vi "ContFindIterationEnd.vi"(11 "Continuous Program in":string[][](array[string])) -> (3 "Array out":i32[][](array[numeric]))   [LabVIEW 2018, in "ContinousLoop.lvlib"]
uses:
  ContinousLoop.lvlib
  <vilib>/regexp/Match Regular Expression.xnode
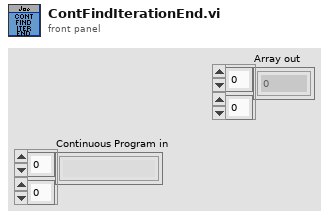
[diagram p1: front panel]
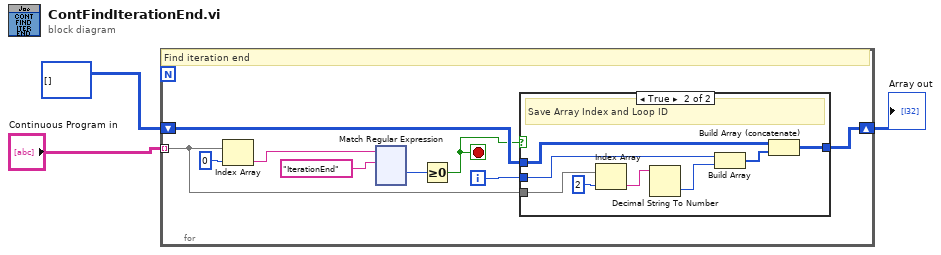
[diagram p0: block diagram]
diagram:
  n1 = for {
    shift-right: [w10] -> w1
    shift-left: i32[][] [] ("Array in") -> [w9]
    tunnel: "Continuous Program in" -> [w6] mode=indexing
    i -> [w5]
    stop <- w4 stop-if-true
    # "Find iteration end"
    n2 = Index Array(array=w6, index=0 ("disabled index (col)")) -> (element=w8:string)
    n3 = xnode "Match Regular Expression"("input string"=w8, "regular expression"="IterationEnd" ("element")) -> ("offset past match"=w11:i32)  [unwired: 4 in, 4 out]
    n4 = Greater Or Equal To 0?(x=w11) -> (x >= 0?=w4:bool)
    n5 = case shown="True" w4 {
      tunnel: [w13 w21] -> w10
      tunnel: w9 -> [w13 w20]
      tunnel: w6 -> [_ w18]
      tunnel: w5 -> [_ w15]
      frame False {
      }
      frame True {
        # "Save Array Index and Loop ID"
        n6 = Index Array(array=w18, index=2 ("disabled index (col)")) -> (element=w17:string)
        n7 = Decimal String To Number(string=w17) -> (number=w16:i32)  [unwired: 2 in, 1 out]
        n8 = Build Array(w15, w16) -> (w14:i32[])
        n9 = Build Array (concatenate)(w20, w14) -> (w21:i32[][])
      }
    }
  }
  "Array out" <- w1
